vi "Get Default White Balance Matrix.vi"(8 "error in (no error)":errorcluster, 11 "TLCamera reference":refnum<k24>) -> (0 "error out":errorcluster, 2 "Default White Balance Matrix":sgl[](array[numeric]), 3 "TLCamera reference out":refnum<k24>)   [LabVIEW 2015]
uses:
  C:/code/Host/Installer/Scientific Camera Interfaces/LabVIEW/32_bit/Library_X86/Thorlabs.TSI.TLCameraInterfaces.dll
  code/Host/Installer/Scientific Camera Interfaces/LabVIEW/32_bit/Library_X86/Thorlabs.TSI.TLCameraInterfaces.dll
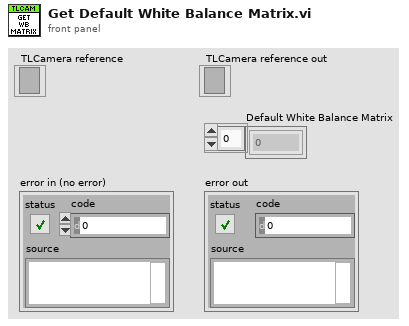
[diagram p1: front panel]
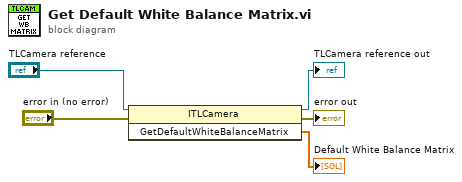
[diagram p0: block diagram]
diagram:
  n1 = invoke class="ITLCamera" method="GetDefaultWhiteBalanceMatrix"(reference="TLCamera reference", error in="error in (no error)") -> (reference out=→"TLCamera reference out":refnum<k24>, error out=→"error out":errorcluster, "GetDefaultWhiteBalanceMatrix"=→"Default White Balance Matrix":sgl[])  [unwired: 1 in]
